vi "SWERVE_TRAJECTORY_DASH_WRITE.vi"   [LabVIEW 2023]
uses:
  <vilib>/Rock Robotics/Network Tables/NT Write Numeric Array.vi
  SWERVE_TRAJECTORY_GLOBALS.vi
  <vilib>/Rock Robotics/Network Tables/NT Write Number.vi
  <vilib>/Rock Robotics/Network Tables/NT Write Boolean.vi
types:
  T1 = typedef "Trajectory_Library.lvlib/SWERVE_DRIVE_ODOMETRY.ctl" = cluster{"POSE":T2, "GyroOffset":T4, "PreviousAngle":T4, "PrevModulePositions":T5[], "NumModules":i32}
  T2 = typedef "Trajectory_Library.lvlib/POSE2D.ctl" = cluster{"TRANSLATION":T3, "ROTATION":T4}
  T3 = typedef "Trajectory_Library.lvlib/TRANSLATION2D.ctl" = cluster{"X":dbl, "Y":dbl}
  T4 = typedef "Trajectory_Library.lvlib/ROTATION2D.ctl" = cluster{"VALUE":dbl, "COS":dbl, "SIN":dbl}
  T5 = typedef "Trajectory_Library.lvlib/SWERVE_DRIVE_MODULE_POSITION.ctl" = cluster{"Distance":dbl, "Angle":T4, "P":bool}
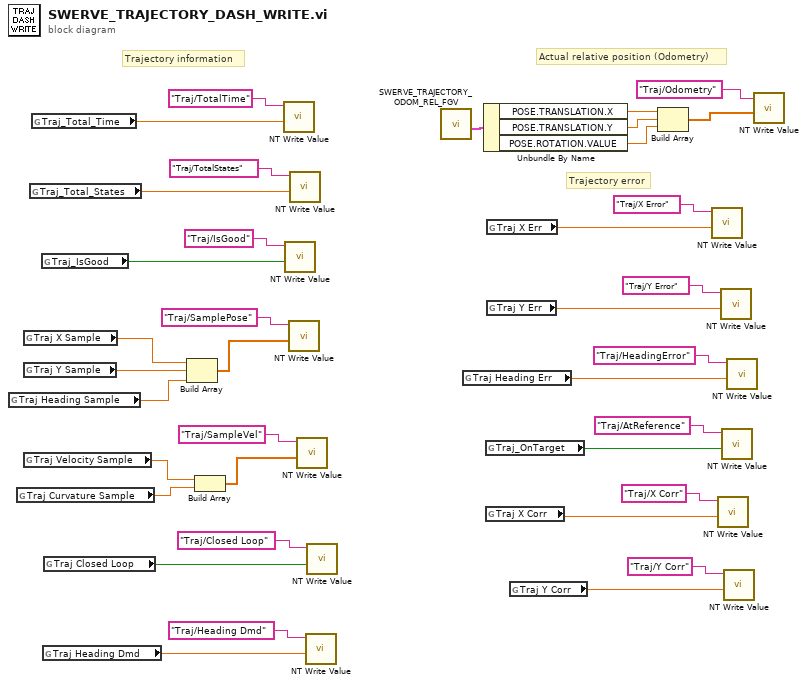
[diagram p0: block diagram]
diagram:
  # "Trajectory information"
  # "Actual relative position (Odometry)"
  # "Trajectory error"
  n1 = global read "SWERVE_TRAJECTORY_GLOBALS.vi" "Traj Heading Sample"() -> (w11:dbl)
  n2 = global read "SWERVE_TRAJECTORY_GLOBALS.vi" "Traj Curvature Sample"() -> (w9:dbl)
  n3 = global read "SWERVE_TRAJECTORY_GLOBALS.vi" "Traj X Sample"() -> (w13:dbl)
  n4 = global read "SWERVE_TRAJECTORY_GLOBALS.vi" "Traj Y Sample"() -> (w12:dbl)
  n5 = global read "SWERVE_TRAJECTORY_GLOBALS.vi" "Traj Velocity Sample"() -> (w10:dbl)
  n6 = global read "SWERVE_TRAJECTORY_GLOBALS.vi" "Traj_Total_States"() -> (w15:dbl)
  n7 = global read "SWERVE_TRAJECTORY_GLOBALS.vi" "Traj_Total_Time"() -> (w14:dbl)
  n8 = global read "SWERVE_TRAJECTORY_GLOBALS.vi" "Traj_IsGood"() -> (w16:bool)
  n9 = global read "SWERVE_TRAJECTORY_GLOBALS.vi" "Traj Heading Dmd"() -> (w7:dbl)
  n10 = global read "SWERVE_TRAJECTORY_GLOBALS.vi" "Traj Closed Loop"() -> (w8:bool)
  n11 = Build Array(w13, w12, w11) -> (w31:dbl[])
  n12 = Build Array(w10, w9) -> (w33:dbl[])
  n13 = call-poly <vilib>:"NT Write Value.vi"("value"=w14, "name"="Traj/TotalTime" ("Name")) -> ()  [unwired: 9 in, 1 out]
  n14 = call-poly <vilib>:"NT Write Value.vi"("value"=w16, "name"="Traj/IsGood" ("Name")) -> ()  [unwired: 9 in, 1 out]
  n15 = call-poly <vilib>:"NT Write Value.vi"("value"=w31, "name"="Traj/SamplePose" ("Name")) -> ()  [unwired: 9 in, 1 out]
  n16 = call-poly <vilib>:"NT Write Value.vi"("value"=w15, "name"="Traj/TotalStates" ("Name")) -> ()  [unwired: 9 in, 1 out]
  n17 = call-poly <vilib>:"NT Write Value.vi"("value"=w33, "name"="Traj/SampleVel" ("Name")) -> ()  [unwired: 9 in, 1 out]
  n18 = call-poly <vilib>:"NT Write Value.vi"("value"=w7, "name"="Traj/Heading Dmd" ("Name")) -> ()  [unwired: 9 in, 1 out]
  n19 = call-poly <vilib>:"NT Write Value.vi"("value"=w8, "name"="Traj/Closed Loop" ("Name")) -> ()  [unwired: 9 in, 1 out]
  n20 = call "SWERVE_TRAJECTORY_ODOM_REL_FGV.vi"() -> ("out SWERVE_DRIVE_ODOMETRY"=w26:T1)  [unwired: 11 in]
  n21 = global read "SWERVE_TRAJECTORY_GLOBALS.vi" "Traj Heading Err"() -> (w4:dbl)
  n22 = Unbundle By Name(w26) -> ("POSE.TRANSLATION.X"=w27:dbl, "POSE.TRANSLATION.Y"=w28:dbl, "POSE.ROTATION.VALUE"=w29:dbl)
  n23 = global read "SWERVE_TRAJECTORY_GLOBALS.vi" "Traj_OnTarget"() -> (w3:bool)
  n24 = global read "SWERVE_TRAJECTORY_GLOBALS.vi" "Traj X Corr"() -> (w1:dbl)
  n25 = global read "SWERVE_TRAJECTORY_GLOBALS.vi" "Traj X Err"() -> (w5:dbl)
  n26 = global read "SWERVE_TRAJECTORY_GLOBALS.vi" "Traj Y Err"() -> (w6:dbl)
  n27 = global read "SWERVE_TRAJECTORY_GLOBALS.vi" "Traj Y Corr"() -> (w2:dbl)
  n28 = Build Array(w27, w28, w29) -> (w24:dbl[])
  n29 = call-poly <vilib>:"NT Write Value.vi"("value"=w5, "name"="Traj/X Error" ("Name")) -> ()  [unwired: 9 in, 1 out]
  n30 = call-poly <vilib>:"NT Write Value.vi"("value"=w1, "name"="Traj/X Corr" ("Name")) -> ()  [unwired: 9 in, 1 out]
  n31 = call-poly <vilib>:"NT Write Value.vi"("value"=w6, "name"="Traj/Y Error" ("Name")) -> ()  [unwired: 9 in, 1 out]
  n32 = call-poly <vilib>:"NT Write Value.vi"("value"=w3, "name"="Traj/AtReference" ("Name")) -> ()  [unwired: 9 in, 1 out]
  n33 = call-poly <vilib>:"NT Write Value.vi"("value"=w2, "name"="Traj/Y Corr" ("Name")) -> ()  [unwired: 9 in, 1 out]
  n34 = call-poly <vilib>:"NT Write Value.vi"("value"=w4, "name"="Traj/HeadingError" ("Name")) -> ()  [unwired: 9 in, 1 out]
  n35 = call-poly <vilib>:"NT Write Value.vi"("value"=w24, "name"="Traj/Odometry" ("Name")) -> ()  [unwired: 9 in, 1 out]
